vi "Multiple OPC Items Monitor.vi"() -> ()   [LabVIEW 2012]
doc: "This VI reads multiple OPC items at one time. Specify which items you want to read or use the predetermined list of items. The predetermined list of items specifies items from the National Instruments.OPCDemo server, which has been installed on your machine."
panel:
  out "Chart":dbl[][](graph)
  out "Error reading items":bool
  out "Time out from server":bool
  in  "Select Items":bool=TRUE
  in  "Number of items to select":i8=3
  in  "stop":bool
  # "Select Help»Show Context Help and move the cursor \nover the VI icon to display help for this VI."
  # "Predetermined\nlist of items"
  # "Select\nitems"
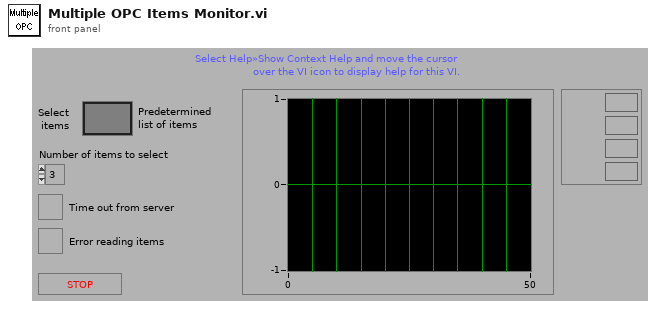
[diagram p1: front panel]
types:
  T1 = enum16{"Read", "Write", "ReadWrite", "BufferedRead", "BufferedReadWrite"}
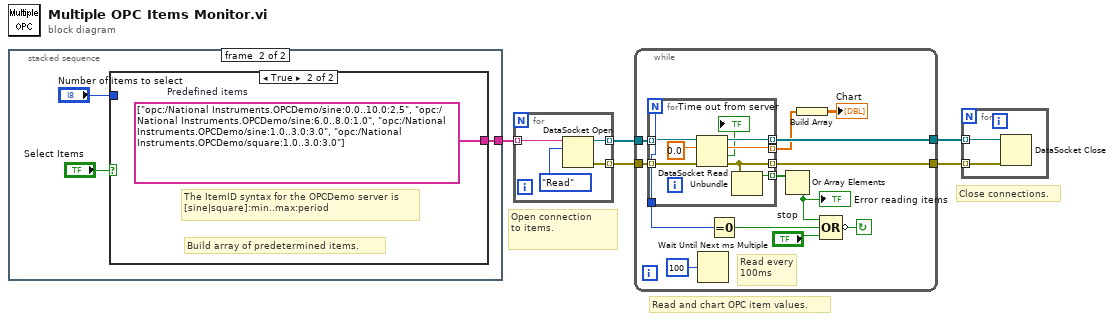
[diagram p0: block diagram]
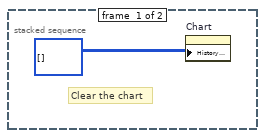
[diagram p2: hidden frame]
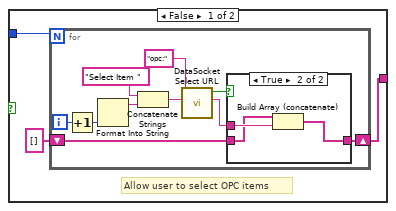
[diagram p3: hidden frame]
diagram:
  # "Read and chart OPC item values."
  # "Close connections."
  # "Open connection \nto items."
  n1 = stacked-sequence {
    tunnel: [_ w9] -> w5
    frame #0 {
      # "Clear the chart"
      n2 = property on="Chart" class="WFChart (strict)"("History Data"=i32[][] [] ("Array Constant")) -> ()  [unwired: 2 in, 2 out]
    }
    frame #1 {
      n3 = case shown="True" "Select Items" {
        tunnel: [w12 w27] -> w9
        tunnel: "Number of items to select" -> [w10 _]
        frame False {
          # "Allow user to select OPC items"
          n4 = for {
            N: w10 -> [_]
            shift-right: [w20] -> w12
            shift-left: string[] [] ("Array Constant") -> [w21]
            i -> [w17]
            n5 = Increment(x=w17) -> (x+1=w15:i32)
            n6 = Format Into String(w15) -> (resulting string=w16:string)  [unwired: 3 in, 1 out]
            n7 = Concatenate Strings("Select Item ", w16) -> (w19:string)
            n8 = call <vilib>:"DataSocket Select URL.vi"("Title (Select URL)"=w19, "StartURL (empty)"="opc:" ("URL")) -> ("URL"=w14:string, "URL Selected"=w22:bool)  [unwired: 1 in, 7 out]
            n9 = case shown="True" w22 {
              tunnel: w14 -> [_ w26]
              tunnel: w21 -> [w23 w24]
              tunnel: [w23 w25] -> w20
              frame False {
                # "If no URL is selected, don't add the item to the item array."
              }
              frame True {
                n10 = Build Array (concatenate)(w24, w26) -> (w25:string[])
              }
            }
          }
        }
        frame True {
          w27 = string[] ["opc:/National Instruments.OPCDemo/sine:0.0..10.0:2.5", "opc:/National Instruments.OPCDemo/sine:6.0..8.0:1.0", "opc:/National Instruments.OPCDemo/sine:1.0..3.0:3.0", "opc:/National Instruments.OPCDemo/square:1.0..3.0:3.0"]  # Predefined items
          # "The ItemID syntax for the OPCDemo server is\n[sine|square]:min..max:period"
          # "Build array of predetermined items."
        }
      }
    }
  }
  n11 = for {
    tunnel: w5 -> [w31] mode=indexing
    tunnel: [w30] -> w4 mode=indexing
    tunnel: [w29] -> w2 mode=indexing
    n12 = DataSocket Open(10:T1."Read" ("mode"), 11:w31) -> (0:w29:errorcluster, 3:w30:refnum<k13>)  [unwired: 1 in, 1 out]
  }
  n13 = while {
    tunnel: [w38] -> w1
    tunnel: w2 -> [w39]
    tunnel: [w43] -> w3
    tunnel: w4 -> [w44]
    stop <- w35 continue-if-true
    # "Read every\n100ms"
    n14 = for {
      N -> [w52]
      tunnel: w44 -> [w49] mode=indexing
      tunnel: [w53] -> w43 mode=indexing
      tunnel: [w52] -> w42
      tunnel: w39 -> [w48] mode=indexing
      tunnel: [w46] -> w41 mode=indexing
      tunnel: [w51] -> w38 mode=indexing
      tunnel: [w50] -> w37 mode=indexing
      n15 = DataSocket Read(8:w48, 10:0.0, 11:w49) -> (0:w51:errorcluster, 1:→"Time out from server":bool, 2:w46:dbl, 3:w53:refnum<k13>)  [unwired: 5 out]
      n16 = Unbundle(w51) -> ("status"=w50:bool)  [unwired: 2 out]
    }
    n17 = Wait Until Next ms Multiple(millisecond multiple=u32 100) -> ()  [unwired: 1 out]
    n18 = Equal To 0?(x=w42) -> (x = 0?=w36:bool)
    n19 = Or Array Elements(Boolean array=w37) -> (logical OR=w33:bool)
    "Error reading items" <- w33
    n20 = Build Array(w41) -> (→"Chart":dbl[][])
    n21 = Compound Arithmetic op=OR(w33, w36, "stop") -> (invert w35:bool)
  }
  n22 = for {
    tunnel: w3 -> [w55] mode=indexing
    tunnel: w1 -> [w54] mode=indexing
    n23 = DataSocket Close(8:w54, 11:w55) -> ()  [unwired: 3 out]
  }
